vi "AlliGator Get Python Script Function List.vi"(8 "error in (no error)":errorcluster, 11 "File Path":path) -> (0 "error out":errorcluster, 1 "Parent Menu Locations":string[](array[string]), 3 "Array of Python Functions Info":T1[](array[typedef]))   [LabVIEW 2021, in "AlliGator Python Plugins.lvlib"]
doc: "Extracts list of python plugin functions and their information from python script."
uses:
  AlliGator Python Plugins.lvlib
  AlliGator Python Function Information.ctl
  AlliGator Python Function Parameter Definition.ctl
  AlliGator Python Function Output Definition.ctl
  AlliGator Python Plugin Target Type.ctl
  <userlib>/_OpenG.lib/string/string.llb/openg_string.lvlib
  Strings/Strings.lvlib
  Error/Error.lvlib
panel:
  # "see the AlliGator License on the block diagram (Ctrl+E or Window:Show Block Diagram)"
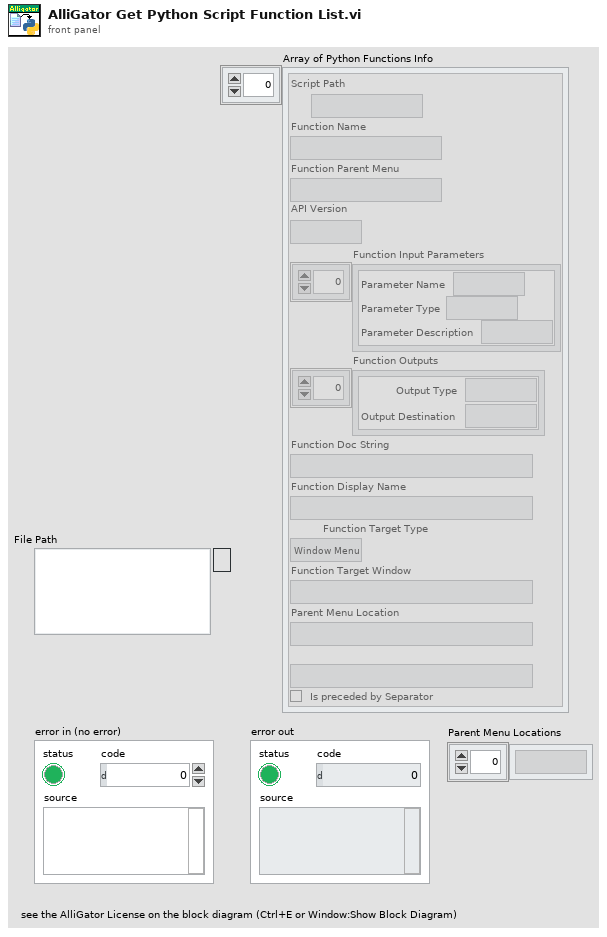
[diagram p1: front panel]
types:
  T1 = typedef "AlliGator Python Plugins.lvlib/AlliGator Python Function Information.ctl" = cluster{"Script Path":path, "Function Name":string, "Function Parent Menu":string, "API Version":string, "Function Input Parameters":T2[], "Function Outputs":T3[], "Function Doc String":string, "Function Display Name":string, "Function Target Type":T4, "Function Target Window":string, "Parent Menu Location":string, "Item Menu Tag":string, "Is preceded by Separator":bool}
  T2 = typedef "AlliGator Python Plugins.lvlib/AlliGator Python Function Parameter Definition.ctl" = cluster{"Parameter Name":string, "Parameter Type":string, "Parameter Description":string}
  T3 = typedef "AlliGator Python Plugins.lvlib/AlliGator Python Function Output Definition.ctl" = cluster{"Output Type":string, "Output Destination":string}
  T4 = typedef "AlliGator Python Plugins.lvlib/AlliGator Python Plugin Target Type.ctl" = enum16{"Undefined", "Window Menu", "Object Menu"}
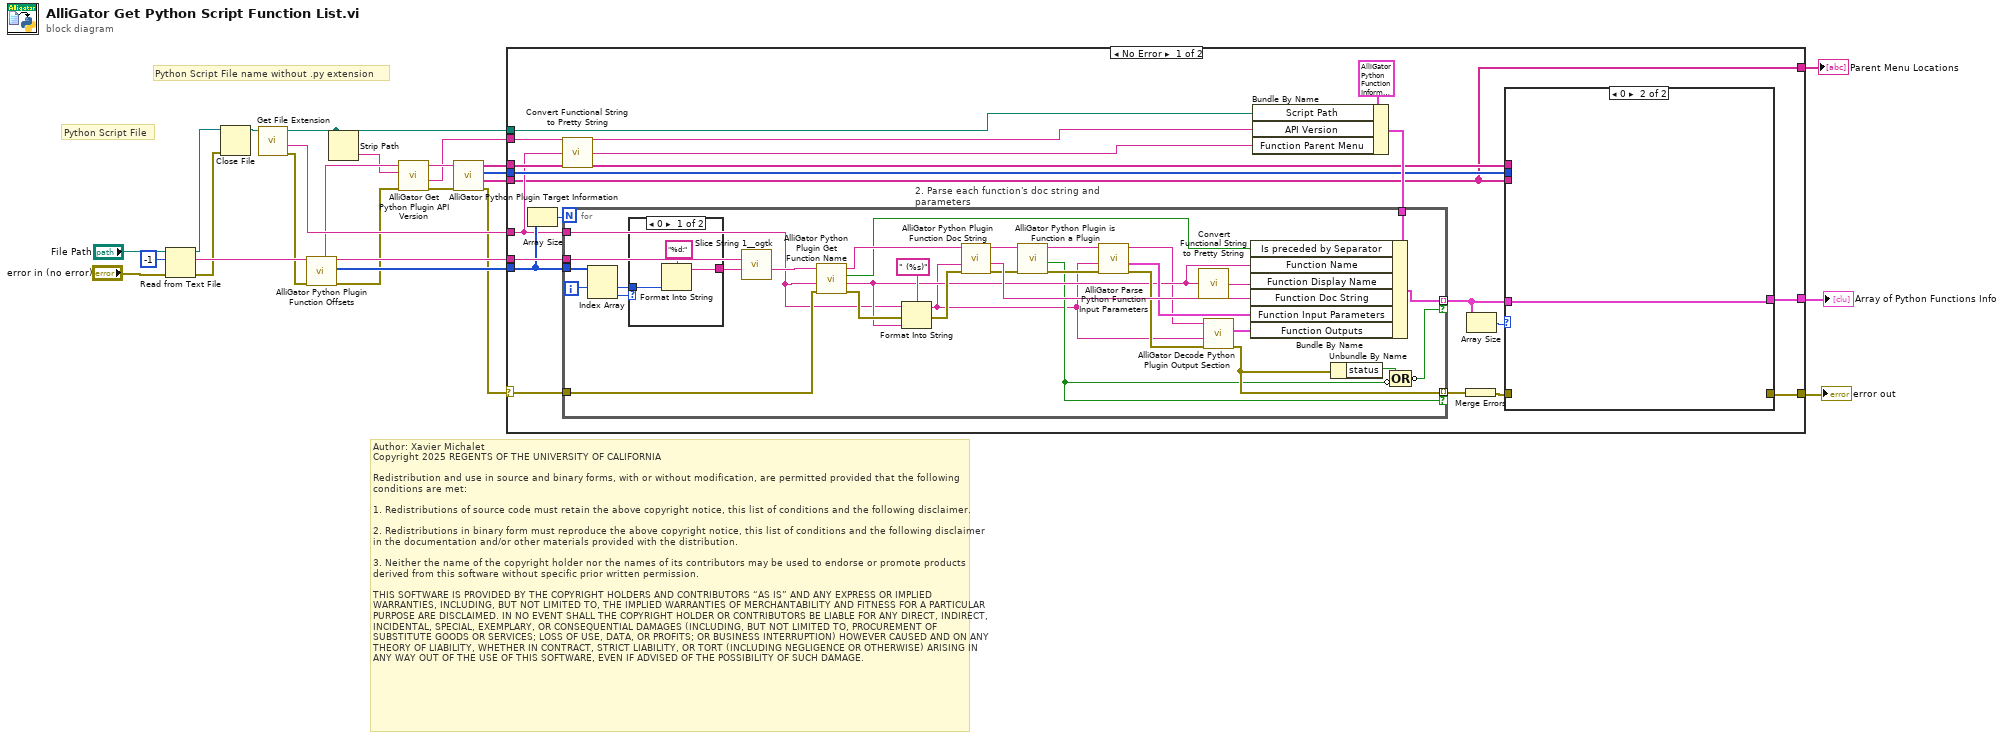
[diagram p0: block diagram]
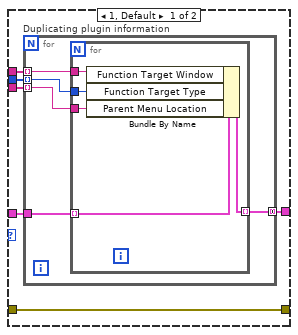
[diagram p2: hidden frame]
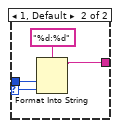
[diagram p3: hidden frame]
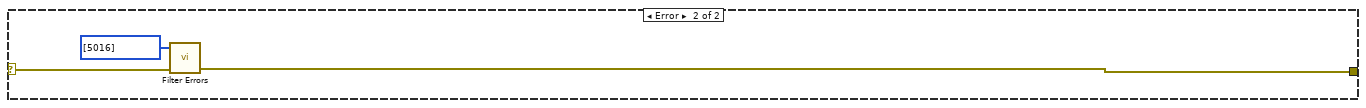
[diagram p4: hidden frame]
diagram:
  # "Author: Xavier Michalet\nCopyright 2025 REGENTS OF THE UNIVERSITY OF CALIFORNIA\n\nRedistribution and use in source and binary forms, with or without modification, are permitted provided that the following conditions are met:\n\n1. Redistributions of source code must retain the above copyright notice, this list of conditions and the following disclaimer.\n\n2. Redistributions in binary form must reproduce the above copyright notice, this list of conditions and the following disclaimer in the documentation and/or other materials provided with the distribution.\n\n3. Neither the name of the copyright holder nor the names of its contributors may be used to endorse or promote products derived from this software without specific prior written permission.\n\nTHIS SOFTWARE IS PROVIDED BY THE COPYRIGHT HOLDERS AND CONTRIBUTORS “AS IS” AND ANY EXPRESS OR IMPLIED WARRANTIES, INCLUDING, BUT NOT LIMITED TO, THE IMPLIED WARRANTIES OF MERCHANTABILITY AND FITNESS FOR A PARTICULAR PURPOSE ARE DISCLAIMED. IN NO EVENT SHALL THE COPYRIGHT HOLDER OR CONTRIBUTORS BE LIABLE FOR ANY DIRECT, INDIRECT, INCIDENTAL, SPECIAL, EXEMPLARY, OR CONSEQUENTIAL DAMAGES (INCLUDING, BUT NOT LIMITED TO, PROCUREMENT OF SUBSTITUTE GOODS OR SERVICES; LOSS OF USE, DATA, OR PROFITS; OR BUSINESS INTERRUPTION) HOWEVER CAUSED AND ON ANY THEORY OF LIABILITY, WHETHER IN CONTRACT, STRICT LIABILITY, OR TORT (INCLUDING NEGLIGENCE OR OTHERWISE) ARISING IN ANY WAY OUT OF THE USE OF THIS SOFTWARE, EVEN IF ADVISED OF THE POSSIBILITY OF SUCH DAMAGE."
  # "Python Script File name without .py extension"
  # "Python Script File"
  n1 = Read from Text File(file (use dialog)="File Path", count=-1, error in="error in (no error)") -> (refnum out=w23:refnum<file>, text=w20:string, error out=w17:errorcluster)  [unwired: 1 in, 1 out]
  n2 = Close File(refnum=w23, error in=w17) -> (path=w21:path)  [unwired: 1 out]
  n3 = call <vilib>:"Get File Extension.vi"("file"=w21) -> ("error out"=w16:errorcluster, "filename without extension"=w15:string, "dup file"=w2:path)  [unwired: 6 in, 2 out]
  n4 = call "AlliGator Python Plugin Function Offsets.vi"("Error In"=w16, "String in"=w20) -> ("Error Out"=w13:errorcluster, "Function Offsets"=w18:i32[], "String in (dup)"=w19:string, "Script Header"=w14:string)  [unwired: 6 in]
  n5 = Strip Path(path=w2) -> (name=w1:string)  [unwired: 1 out]
  n6 = call "AlliGator Get Python Plugin API Version.vi"("error in (no error)"=w13, "Source"=w1, "Script Header"=w14) -> ("error out"=w5:errorcluster, "API Version"=w3:string, "Script Header - Version"=w4:string)  [unwired: 6 in]
  n7 = call "AlliGator Python Plugin Target Information.vi"("error in (no error)"=w5, "Script Header"=w4) -> ("error out"=w12:errorcluster, "Parent Menu Locations"=w8:string[], "Function Target Types"=w9:T4[], "Function Target Windows"=w10:string[])  [unwired: 6 in]
  n8 = case shown="No Error" w12 {
    selector: w12 -> [w38 w103]
    tunnel: w2 -> [w42 _]
    tunnel: w19 -> [w41 _]
    tunnel: w18 -> [w40 _]
    tunnel: w15 -> [w31 _]
    tunnel: [w29 w101] -> w11
    tunnel: w10 -> [w36 _]
    tunnel: w9 -> [w35 _]
    tunnel: w8 -> [w27 _]
    tunnel: [w34 _] -> w7
    tunnel: [w27 _] -> w6
    tunnel: w3 -> [w26 _]
    frame No Error {
      n9 = Array Size(array=w40) -> (size(s)=w39:i32)
      n10 = call "Convert Functional String to Pretty String.vi"("Functional Name"=w31) -> ("Pretty Name"=w28:string)  [unwired: 4 in]
      n11 = Bundle By Name(cluster=T1 {"Script Path"=path "", "Function Name"="", "Function Parent Menu"="", "API Version"="", "Function Input Parameters"=[], "Function Outputs"=[], "Function Doc String"="", "Function Display Name"="", "Function Target Type"=enum."Window Menu", "Function Target Window"="", "Parent Menu Location"="", "Item Menu Tag"="", "Is preceded by Separator"=FALSE} ("Array of Python Functions Info"), "Script Path"=w42, "API Version"=w26, "Function Parent Menu"=w28) -> (w43:T1)
      n12 = for "2. Parse each function's doc string and parameters" {
        N: w39 -> [_]
        tunnel: w41 -> [w91]
        tunnel: w43 -> [w93]
        tunnel: [w92] -> w33 mode=indexing if=w70
        tunnel: w40 -> [w90]
        tunnel: w31 -> [w62]
        tunnel: w38 -> [w83]
        tunnel: [w72] -> w37 mode=indexing if=w66
        i -> [w89]
        n13 = Index Array(array=w90, index #1=w89) -> (element #1=w88:i32, element #2=w87:i32)  [unwired: 1 in]
        n14 = case shown="0" w87 {
          selector: w87 -> [_ w99]
          tunnel: w88 -> [w96 w100]
          tunnel: [w94 w97] -> w86
          frame 0 {
            n15 = Format Into String(format string="%d:", w96) -> (resulting string=w94:string)  [unwired: 2 in, 1 out]
          }
          frame 1, Default {
            n16 = Format Into String(format string="%d:%d", w100, w99) -> (resulting string=w97:string)  [unwired: 2 in, 1 out]
          }
        }
        n17 = call <userlib>:"Slice String 1__ogtk.vi"("Subset (i:j)"=w86, "String"=w91) -> ("Substring (String[i:j])"=w85:string)  [unwired: 7 in]
        n18 = call "AlliGator Python Plugin Get Function Name.vi"("Error In"=w83, "Source"=w62, "String in"=w85) -> ("Error Out"=w81:errorcluster, "function_name"=w69:string, "Is preceded by Separator"=w65:bool, "String out"=w84:string)  [unwired: 5 in]
        n19 = Format Into String(format string=" (%s)", initial string=w62, error in=w81, w69) -> (resulting string=w63:string, error out=w80:errorcluster)
        n20 = call "AlliGator Python Plugin Function Doc String.vi"("Error In"=w80, "Source"=w63, "String in"=w84) -> ("Error Out"=w77:errorcluster, "Doc String"=w78:string, "String out"=w82:string)  [unwired: 6 in]
        n21 = call "AlliGator Python Plugin is Function a Plugin.vi"("Error In"=w77, "String in"=w82) -> ("Error Out"=w76:errorcluster, "Is AlliGator Python Plugin?"=w66:bool, "String out"=w75:string)  [unwired: 7 in]
        n22 = call "AlliGator Parse Python Function Input Parameters.vi"("Error In"=w76, "Source"=w63, "Input String"=w75) -> ("Error Out"=w74:errorcluster, "Function Input Parameters"=w73:T2[], "Output string"=w64:string)  [unwired: 6 in]
        n23 = call "Convert Functional String to Pretty String.vi"("Functional Name"=w69) -> ("Pretty Name"=w68:string)  [unwired: 4 in]
        n24 = call "AlliGator Decode Python Plugin Output Section.vi"("error in (no error)"=w74, "Source"=w63, "Input String"=w64) -> ("error out"=w72:errorcluster, "Function Outputs"=w67:T3[])  [unwired: 6 in, 1 out]
        n25 = Bundle By Name(cluster=w93, "Is preceded by Separator"=w65, "Function Name"=w69, "Function Display Name"=w68, "Function Doc String"=w78, "Function Input Parameters"=w73, "Function Outputs"=w67) -> (w92:T1)
        n26 = Unbundle By Name(w72) -> ("status"=w71:bool)
        n27 = Compound Arithmetic op=OR(w71, invert w66) -> (invert w70:bool)
      }
      n28 = Merge Errors(w37) -> (w30:errorcluster)
      n29 = Array Size(array=w33) -> (size(s)=w32:i32)
      n30 = case shown="0" w32 {
        tunnel: w36 -> [w48 _]
        tunnel: w35 -> [w50 _]
        tunnel: w27 -> [w49 _]
        tunnel: w33 -> [w47 w61]
        tunnel: [w46 w61] -> w34
        tunnel: w30 -> [w45 _]
        tunnel: [w45 _] -> w29
        frame 1, Default {
          n31 = for "Duplicating plugin information" {
            tunnel: w50 -> [w53] mode=indexing
            tunnel: w49 -> [w52] mode=indexing
            tunnel: w48 -> [w54] mode=indexing
            tunnel: w47 -> [w55]
            tunnel: [w51] -> w46 mode=concatenating
            n32 = for {
              tunnel: w55 -> [w60] mode=indexing
              tunnel: w54 -> [w59]
              tunnel: w53 -> [w58]
              tunnel: w52 -> [w57]
              tunnel: [w56] -> w51 mode=indexing
              n33 = Bundle By Name(cluster=w60, "Function Target Window"=w59, "Function Target Type"=w58, "Parent Menu Location"=w57) -> (w56:T1)
            }
          }
        }
        frame 0 {
        }
      }
    }
    frame Error {
      n34 = call "Filter Errors.vi"("Filtered Errors"=i32[] [5016], "error in (no error)"=w103) -> ("error out"=w101:errorcluster)  [unwired: 7 in]
    }
  }
  "error out" <- w11
  "Array of Python Functions Info" <- w7
  "Parent Menu Locations" <- w6
